vi "Scan_2.vi"(0 "DMM ref":refnum<visa-resource-name>, 1 "output cluster":cluster{"Timeout":i32, "Channel number":i32}, 2 "P_current_count":i32, 3 "N_current_count":i32, 5 "DMM error":errorcluster, 7 "Current Sense \nResitance Array":dbl[](array[numeric])=[1.0032214, 1.00250644, 1.00234822, 1.0040944, 1.0017711, 1.00229431, 1.00344206, 1.00482066, 1.00381056, 1.00290978, 1.00333016, 1.00367587], 9 "ESP32 ref":refnum<visa-resource-name>, 11 "ESP32 error":errorcluster, 12 "current_mode":u8[](array[numeric])=[0, 0, 0, 0, 0, 0, 0, 0, 0, 0, 0]) -> (4 "DMM ref":refnum<visa-resource-name>, 6 "DMM error":errorcluster, 8 "Measurements":dbl[](array[numeric]), 10 "ESP32 ref":refnum<visa-resource-name>, 13 "Timout?":bool, 14 "Time out count":i32, 15 "ESP32 error":errorcluster)   [LabVIEW 2023]
uses:
  <instrlib>/Agilent 3446X Series/Agilent 3446X Series.lvlib
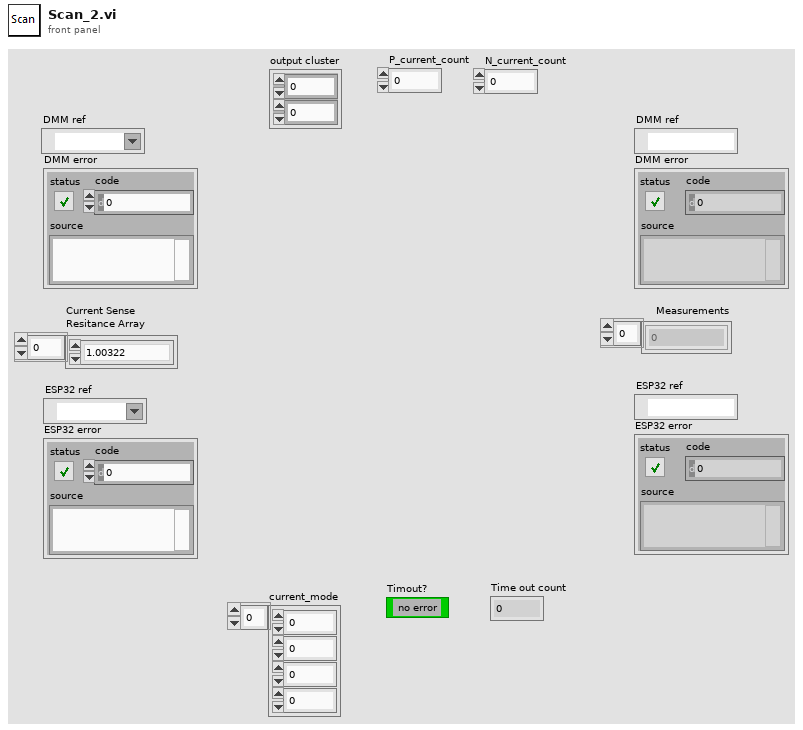
[diagram p1: front panel]
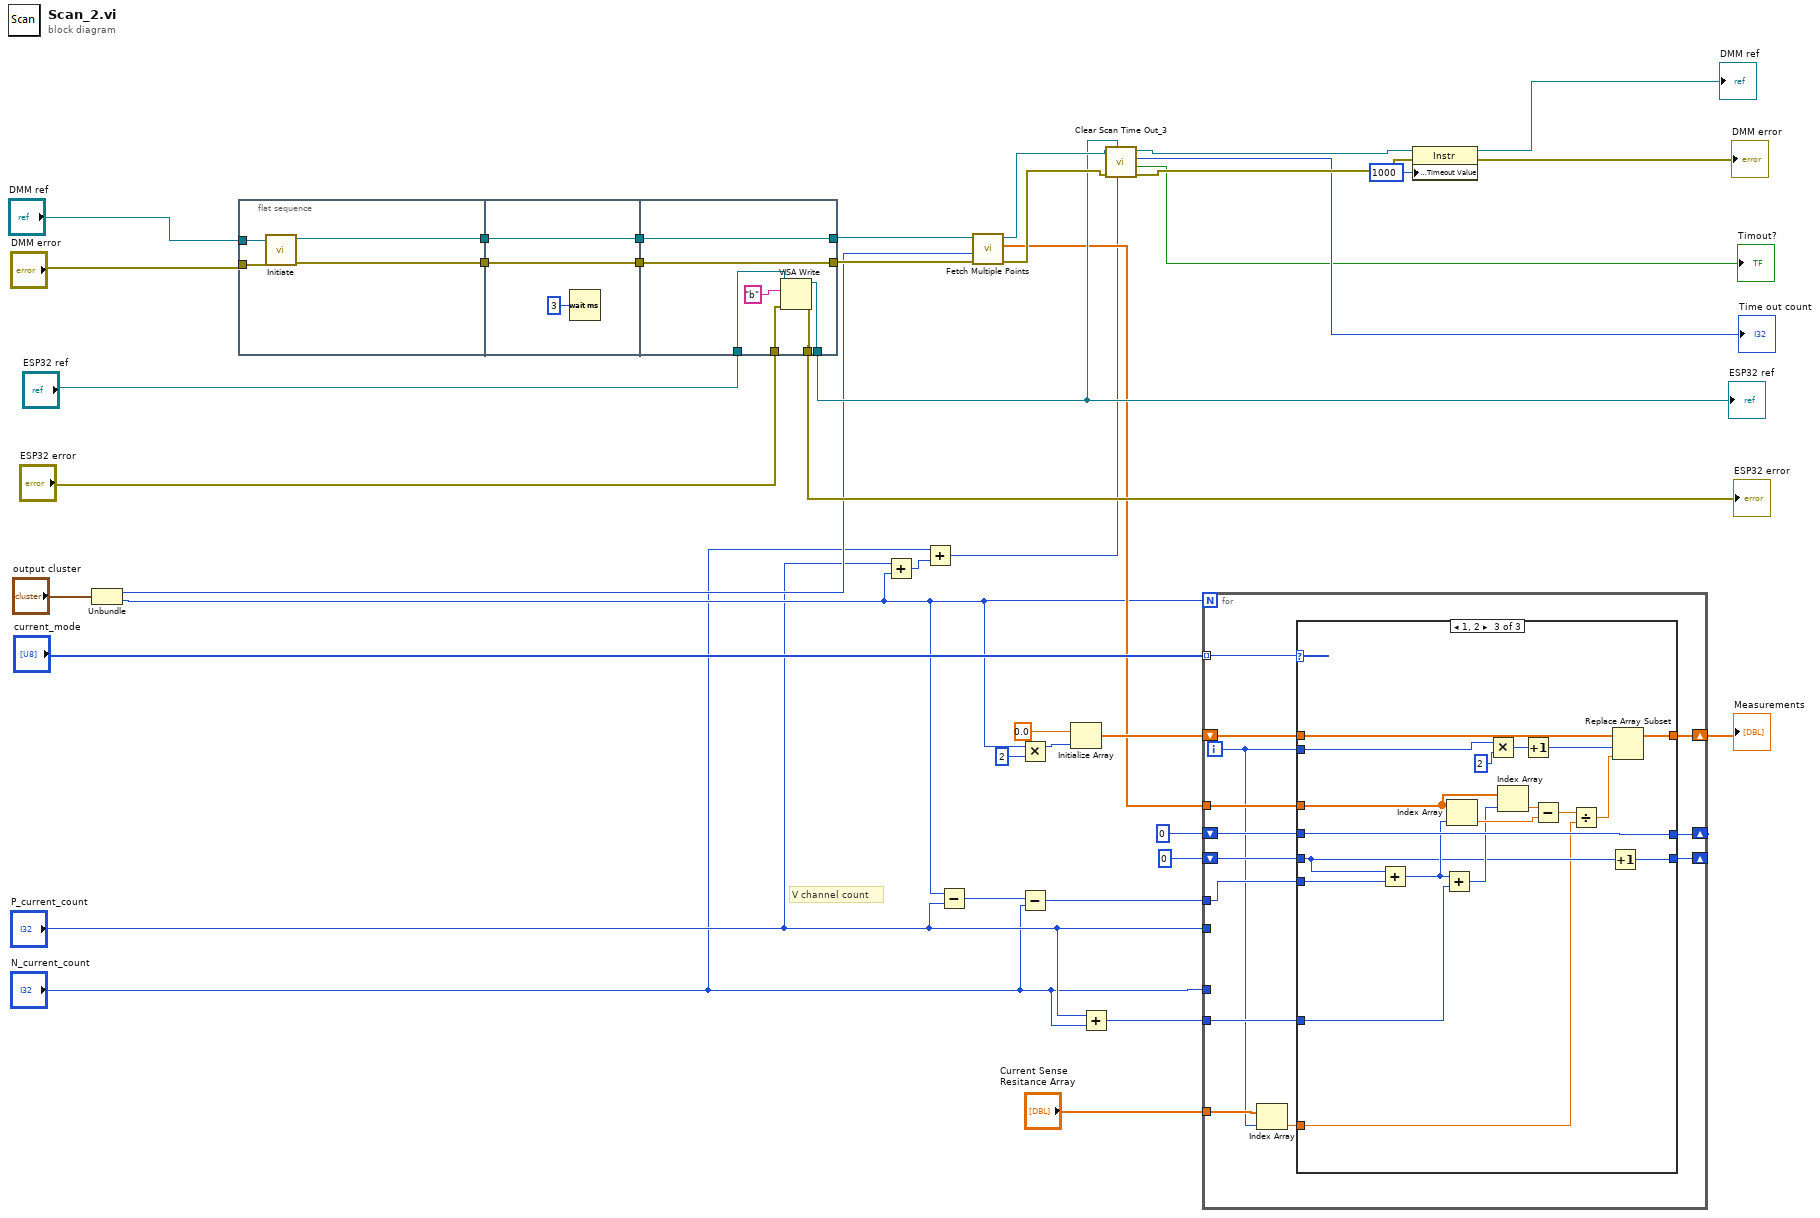
[diagram p0: block diagram]
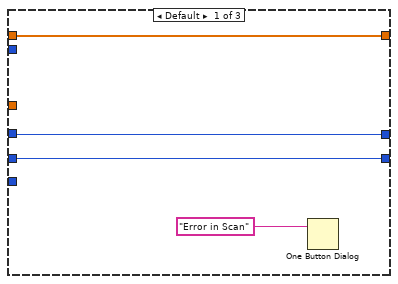
[diagram p2: hidden frame]
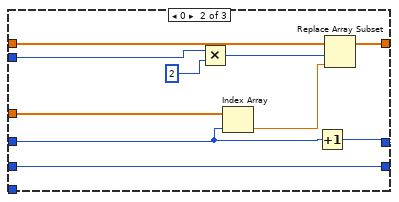
[diagram p3: hidden frame]
diagram:
  # "V channel count"
  n1 = Unbundle("output cluster") -> ("Timeout"=w6:i32, "Channel number"=w5:i32)
  n2 = flat-sequence {
    tunnel: [w45] -> w41
    tunnel: [w44] -> w40
    tunnel: "DMM ref" -> [w43]
    tunnel: "DMM error" -> [w42]
    tunnel: w41 -> [w48]
    tunnel: [w48] -> w39
    tunnel: w40 -> [w47]
    tunnel: [w47] -> w38
    tunnel: w39 -> [w55]
    tunnel: w38 -> [w54]
    tunnel: "ESP32 ref" -> [w53]
    tunnel: "ESP32 error" -> [w52]
    tunnel: [w51] -> w23
    tunnel: [w50] -> w24
    tunnel: [w55] -> w37
    tunnel: [w54] -> w36
    frame #0 {
      n3 = call <instrlib>:"Initiate.vi"("error in (no error)"=w42, "VISA resource name"=w43) -> ("error out"=w45:errorcluster, "VISA resource name out"=w44:refnum<visa-resource-name>)  [unwired: 8 in]
    }
    frame #1 {
      n4 = Wait (ms)(milliseconds to wait=u32 3) -> ()  [unwired: 1 out]
    }
    frame #2 {
      n5 = VISA Write(VISA resource name=w53, write buffer="b" ("data in"), error in (no error)=w52) -> (VISA resource name out=w51:refnum<visa-resource-name>, error out=w50:errorcluster)  [unwired: 1 out]
    }
  }
  n6 = Add(x="P_current_count", y=w5) -> (x+y=w2:i32)
  n7 = Add(x="N_current_count", y=w2) -> (x+y=w1:i32)
  n8 = Subtract(x=w5, y="P_current_count") -> (x-y=w14:i32)
  n9 = call <instrlib>:"Fetch Multiple Points.vi"("error in (no error)"=w37, "Timeout (10000 ms)"=w6, "VISA resource name"=w36) -> ("error out"=w32:errorcluster, "Measurements"=w15:dbl[], "VISA resource name out"=w33:refnum<visa-resource-name>)  [unwired: 1 in, 5 out]
  n10 = Multiply(x=w5, y=2) -> (x*y=w19:i32)
  n11 = Subtract(x=w14, y="N_current_count") -> (x-y=w13:i32)
  n12 = Initialize Array(0.0 ("Measurement"), w19) -> (w17:dbl[])
  n13 = Add(x="P_current_count", y="N_current_count") -> (x+y=w10:i32)
  n14 = call "Clear Scan Time Out_3.vi"("Channel number"=w1, "ESP32 ref"=w23, "error in (no error)"=w32, "VISA Refnum in"=w33) -> ("error out"=w30:errorcluster, "error?"=→"Timout?":bool, "Time out count"=→"Time out count":i32, "VISA Refnum out"=w31:refnum<visa-resource-name>)  [unwired: 3 in, 1 out]
  n15 = for {
    N: w5 -> [_]
    shift-right: [w63] -> w9
    shift-left: w17 -> [w64]
    tunnel: "current_mode" -> [w68] mode=indexing
    tunnel: w15 -> [w67]
    tunnel: "P_current_count" -> [_]
    tunnel: "N_current_count" -> [_]
    tunnel: w13 -> [w60]
    shift-right: [w65] -> _
    shift-left: 0 ("index") -> [w66]
    shift-right: [w61] -> _
    shift-left: 0 ("index") -> [w62]
    tunnel: w10 -> [w59]
    tunnel: "Current Sense \nResitance Array" -> [w58]
    i -> [w57]
    n16 = Index Array(array=w58, index=w57) -> (element=w56:dbl)
    n17 = case shown="1, 2" w68 {
      tunnel: w67 -> [_ w82 w94]
      tunnel: w66 -> [w72 w80 w95]
      tunnel: [w72 w79 w95] -> w65
      tunnel: w57 -> [_ w77 w100]
      tunnel: w64 -> [w71 w78 w101]
      tunnel: [w71 w75 w97] -> w63
      tunnel: w62 -> [w70 w74 w87]
      tunnel: [w70 w74 w86] -> w61
      tunnel: w60 -> [_ _ w91]
      tunnel: w59 -> [_ _ w90]
      tunnel: w56 -> [_ _ w84]
      frame Default {
        n18 = One Button Dialog(message="Error in Scan") -> ()  [unwired: 1 in, 1 out]
      }
      frame 0 {
        n19 = Multiply(x=w77, y=2 ("x")) -> (x*y=w73:i32)
        n20 = Index Array(array=w82, index=w80) -> (element=w81:dbl)
        n21 = Increment(x=w80) -> (x+1=w79:i32)
        n22 = Replace Array Subset(array=w78, new element=w81, index=w73) -> (w75:dbl[])
      }
      frame 1, 2 {
        n23 = Add(x=w87, y=w91) -> (x+y=w89:i32)
        n24 = Add(x=w89, y=w90) -> (x+y=w88:i32)
        n25 = Index Array(array=w94, index=w89) -> (element=w92:dbl)
        n26 = Multiply(x=w100, y=2 ("x")) -> (x*y=w98:i32)
        n27 = Index Array(array=w94, index=w88) -> (element=w93:dbl)
        n28 = Increment(x=w98) -> (x+1=w96:i32)
        n29 = Subtract(x=w93, y=w92) -> (x-y=w85:dbl)
        n30 = Divide(x=w85, y=w84) -> (x/y=w83:dbl)
        n31 = Increment(x=w87) -> (x+1=w86:i32)
        n32 = Replace Array Subset(array=w101, new element=w83, index=w96) -> (w97:dbl[])
      }
    }
  }
  "Measurements" <- w9
  n33 = property class="Instr"(reference=w31, error in=w30, "General Settings:Timeout Value"=u32 1000) -> (reference out=→"DMM ref":refnum<visa-resource-name>, error out=→"DMM error":errorcluster)
  "ESP32 ref" <- w23
  "ESP32 error" <- w24
